vi "CENTRIOD DETECTION BEAMPOINTING.vi"(0 "Refnum in":T6=refnum, 4 "beam detection para":T4={"Filter"=1, "Filter Para"={"X Size"=5, "Y Size"=5, "% Tolerance"=1}, "detection method"=4, "smal para"=[{"Measurement Parameter"=35, "Range Lower Value"=0.0, "Range Upper Value"=500.0, "Range"=TRUE, "Measurement Type"=FALSE}], "Remove small Objects"=TRUE, "Restrict to round Objects"=TRUE} {"smal para"."Measurement Parameter" items=["Center of Mass X", "Center of Mass Y", "First Pixel X", "First Pixel Y", "Bounding Rect Left", "Bounding Rect Top", "Bounding Rect Right", "Bounding Rect Bottom", "Max Feret Diameter Start X", "Max Feret Diameter Start Y", "Max Feret Diameter End X", "Max Feret Diameter End Y", "Max Horiz. Segment Length Left", "Max Horiz. Segment Length Right", "Max Horiz. Segment Length Row", "-", "Bounding Rect Width", "Bounding Rect Height", "Bounding Rect Diagonal", "Perimeter", "Convex Hull Perimeter", "Holes' Perimeter", "Max Feret Diameter", "Equivalent Ellipse Major Axis", "Equivalent Ellipse Minor Axis", "Equivalent Ellipse Minor Axis (Feret)", "Equivalent Rect Long Side", "Equivalent Rect Short Side", "Equivalent Rect Diagonal", "Equivalent Rect Short Side (Feret)", "Average Horiz. Segment Length", "Average Vert. Segment Length", "Hydraulic Radius", "Waddel Disk Diameter", "-", "Area", "Holes' Area", "Particle & Holes' Area", "Convex Hull Area", "Image Area", "-", "Number of Holes", "Number of Horiz. Segments", "Number of Vert. Segments", "-", "Orientation", "Max Feret Diameter Orientation", "-", "% Area/Image Area", "% Area/(Particle & Holes' Area)", "Ratio of Equivalent Ellipse Axes", "Ratio of Equivalent Rect Sides", "-", "Elongation Factor", "Compactness Factor", "Heywood Circularity Factor", "Type Factor", "-", "Sum X", "Sum Y", "Sum XX", "Sum XY", "Sum YY", "Sum XXX", "Sum XXY", "Sum XYY", "Sum YYY", "-", "Moment of Inertia XX", "Moment of Inertia XY", "Moment of Inertia YY", "Moment of Inertia XXX", "Moment of Inertia XXY", "Moment of Inertia XYY", "Moment of Inertia YYY", "Norm. Moment of Inertia XX", "Norm. Moment of Inertia XY", "Norm. Moment of Inertia YY", "Norm. Moment of Inertia XXX", "Norm. Moment of Inertia XXY", "Norm. Moment of Inertia XYY", "Norm. Moment of Inertia YYY", "Hu Moment 1", "Hu Moment 2", "Hu Moment 3", "Hu Moment 4", "Hu Moment 5", "Hu Moment 6", "Hu Moment 7"]; "smal para"."Range Lower Value" format="%.2f"; "smal para"."Range Upper Value" format="%.2f"; "detection method" items=["clustering", "entropy", "metric", "moments", "inter-class variance"]; "Filter" items=["No Filter", "Median Filter", "Low Pass Filter"]}, 5 "error in (no error)":errorcluster) -> (8 "Bounding Rect":T7={"Left"=200.0, "Top"=222.0, "Right"=337.0, "Bottom"=354.0}, 11 "Particle Reports (Pixels)":T8(array[cluster])=[{"Area"=13217.0, "Number of Holes"=0.0, "Bounding Rect"={"Left"=200.0, "Top"=222.0, "Right"=337.0, "Bottom"=354.0}, "Center of Mass"={"X"=269.13989558901415, "Y"=287.03949459030036}, "Orientation"=28.32814462161336, "Dimensions"={"Width"=137.0, "Height"=132.0}}] {"Orientation" format="%.2f"; "Dimensions"."Height" format="%.2f"; "Dimensions"."Width" format="%.2f"; "Center of Mass"."Y" format="%.2f"; "Center of Mass"."X" format="%.2f"; "Bounding Rect"."Bottom" format="%.2f"; "Bounding Rect"."Right" format="%.2f"; "Bounding Rect"."Top" format="%.2f"; "Bounding Rect"."Left" format="%.2f"; "Number of Holes" format="%.2f"; "Area" format="%.2f"}, 13 "Area":dbl=13217.0, 14 "Refnum out":T6, 17 "Number of Particles":i32=1, 18 "Centriod":cluster{"X":dbl, "Y":dbl}={"X"=268.53924560546875, "Y"=286.7691955566406}, 19 "error out":errorcluster)   [LabVIEW 2013]
uses:
  <vilib>/vision/Image Controls.llb/IMAQ Image.ctl
  Ctrs/beam detection.ctl
  <vilib>/vision/Measure.llb/Edge Options.ctl
  <vilib>/vision/Measure.llb/Edge Polarity.ctl
  <vilib>/vision/NI_Vision_Development_Module.lvlib
panel:
  out "Circle Found":bool=TRUE
  in  "Options":T3={"Search  Direction"=1, "Edge Options"={"Edge Polarity"=2, "Kernel Size"=3, "Width"=3, "Minimum Edge Strength"=10.0, "Interpolation Type"=enum."Bilinear Fixed", "Data Processing Method"=enum."Average"}, "Show Search Area"=FALSE, "Show Search Lines"=FALSE, "Show Edges Found"=FALSE, "Show Result"=TRUE, "Search Area Color"=65280, "Search Lines Color"=255, "Edge Locations Color"=16776960, "Result Color"=3079978, "Overlay Group Name"=""} {"Search  Direction" items=["Outside to Inside", "Inside to Outside"]; "Edge Options"."Edge Polarity" items=["All Edges", "Rising Edges", "Falling Edges"]; "Edge Options"."Minimum Edge Strength" format="%.2f"; "Edge Options"."Width" step=2; "Edge Options"."Kernel Size" step=2}
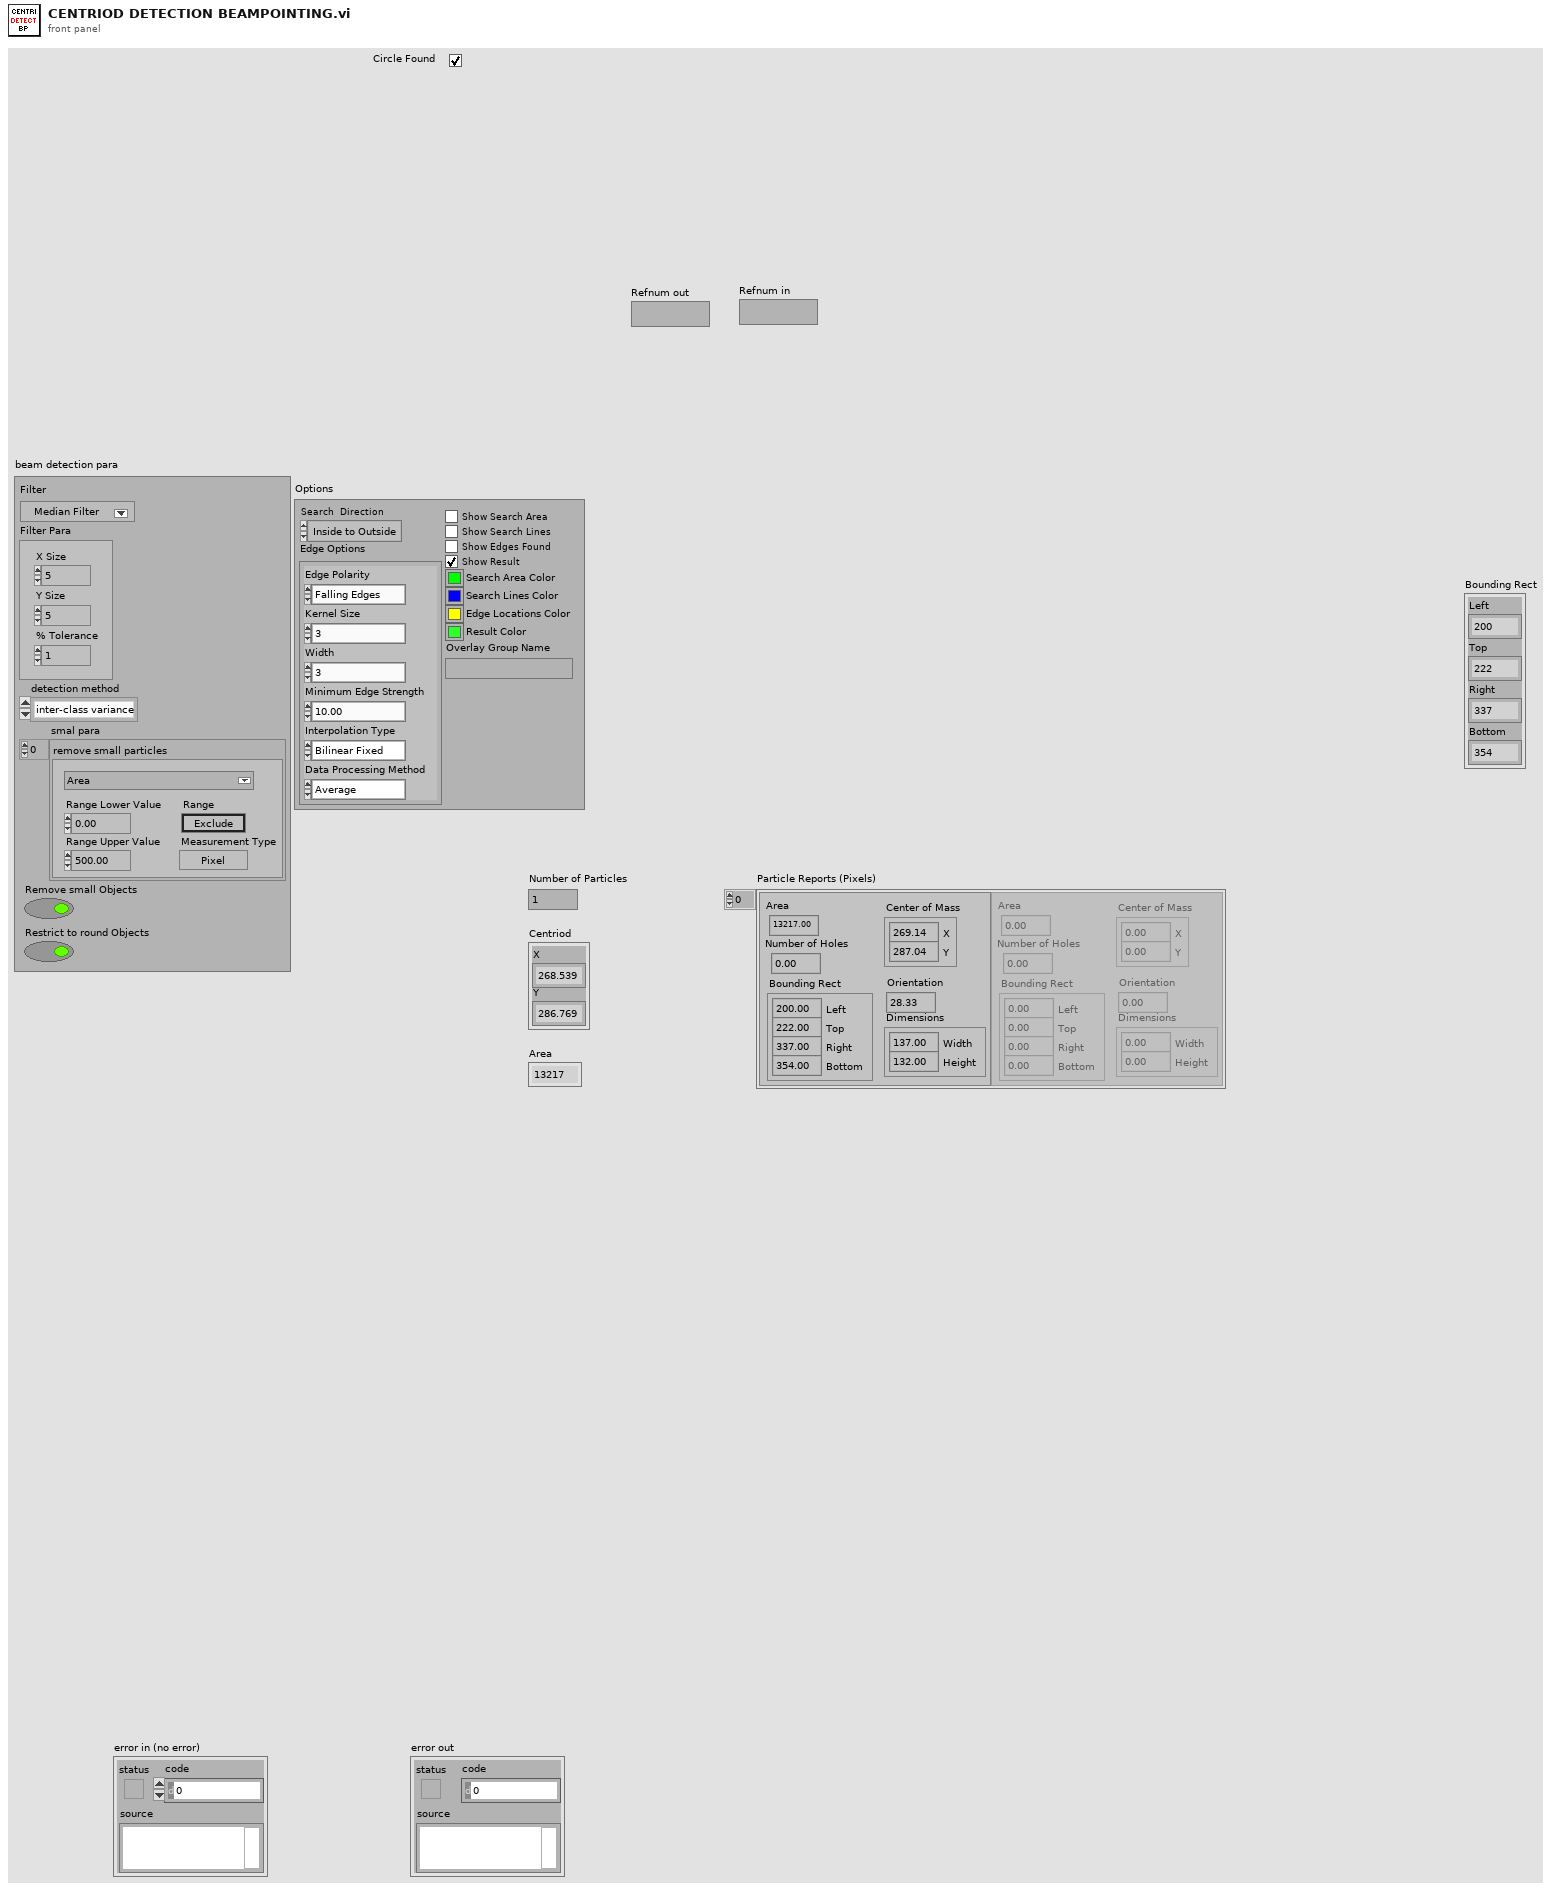
[diagram p1: front panel]
types:
  T1 = typedef "Edge Options.ctl" = cluster{"Edge Polarity":T2, "Kernel Size":u32, "Width":u32, "Minimum Edge Strength":sgl, "Interpolation Type":enum32{"Zero Order", "Bilinear", "Quadratic", "Cubic", "Bilinear Fixed"}, "Data Processing Method":enum32{"Average", "Median"}}
  T2 = typedef "Edge Polarity.ctl" = u32
  T3 = cluster{"Search  Direction":u32, "Edge Options":T1, "Show Search Area":bool, "Show Search Lines":bool, "Show Edges Found":bool, "Show Result":bool, "Search Area Color":u32, "Search Lines Color":u32, "Edge Locations Color":u32, "Result Color":u32, "Overlay Group Name":string}
  T4 = typedef "beam detection.ctl" = cluster{"Filter":u16, "Filter Para":cluster{"X Size":i32, "Y Size":i32, "% Tolerance":i32}, "detection method":i32, "smal para":cluster{"Measurement Parameter":T5, "Range Lower Value":dbl, "Range Upper Value":dbl, "Range":bool, "Measurement Type":bool}[], "Remove small Objects":bool, "Restrict to round Objects":bool}
  T5 = typedef "Particle Parameters" = i32
  T6 = typedef "IMAQ Image.ctl" = refnum<image>
  T7 = cluster{"Left":dbl, "Top":dbl, "Right":dbl, "Bottom":dbl}
  T8 = cluster{"Area":dbl, "Number of Holes":dbl, "Bounding Rect":cluster{"Left":dbl, "Top":dbl, "Right":dbl, "Bottom":dbl}, "Center of Mass":cluster{"X":dbl, "Y":dbl}, "Orientation":dbl, "Dimensions":cluster{"Width":dbl, "Height":dbl}}[]
  T9 = typedef "Image Type" = u32
  T10 = cluster{"X Size":i32, "Y Size":i32, "% Tolerance":i32}
  T11 = typedef "IMAQ Circle" = cluster{"Center X":i32, "Center Y":i32, "Inner Radius":i32, "Outer Radius":i32, "Start Angle":dbl, "End Angle":dbl}
  T12 = cluster{"Measurement Parameter":T5, "Range Lower Value":dbl, "Range Upper Value":dbl, "Range":bool, "Measurement Type":bool}[]
  T13 = cluster{"Area":dbl, "Number of Holes":dbl, "Bounding Rect":cluster{"Left":dbl, "Top":dbl, "Right":dbl, "Bottom":dbl}, "Center of Mass":cluster{"X":dbl, "Y":dbl}, "Orientation":dbl, "Dimensions":cluster{"Width":dbl, "Height":dbl}}
  T14 = typedef "ROI Descriptor" = cluster{"Global Rectangle":i32[], "Contours":cluster{"ID":enum32{"External", "Internal"}, "Type":u32, "Coordinates":i32[]}[]}
  T15 = cluster{"Center (Pixels)":cluster{"X":sgl, "Y":sgl}, "Radius (Pixels)":dbl, "Center (Real-World)":cluster{"X":sgl, "Y":sgl}, "Radius (Real-World)":dbl, "Roundness (Real-World)":dbl, "Average Strength":dbl, "Average SNR (dB)":dbl}
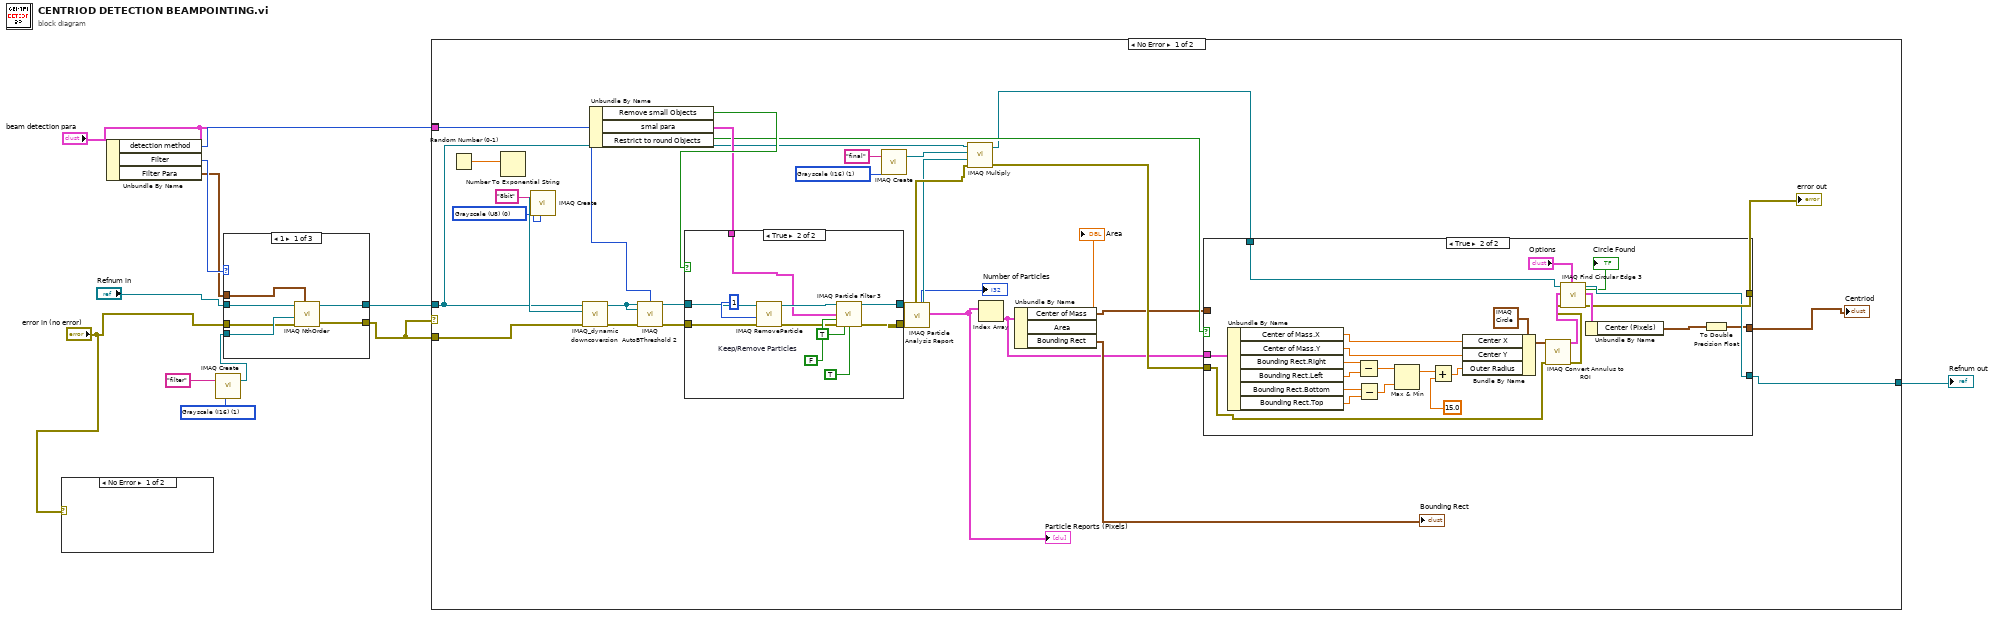
[diagram p0: block diagram]
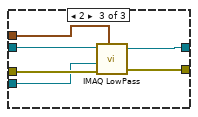
[diagram p7: hidden frame]
diagram:
  w12 = T9 1 items=["Grayscale (U8)", "Grayscale (I16)", "Grayscale (SGL)", "Complex (CSG)", "RGB (U32)", "HSL (U32)", "RGB (U64)", "Grayscale (U16)"] ("Image Type")
  n1 = case shown="No Error" "error in (no error)" {
    frame No Error {
    }
    frame Error {
    }
  }
  n2 = Unbundle By Name("beam detection para") -> ("detection method"=w9:i32, "Filter"=w10:u16, "Filter Para"=w8:T10)
  n3 = call "IMAQ Create"("Image Name"="filter", "Image Type"=w12) -> ("New Image"=w11:T6)  [unwired: 3 in, 1 out]
  n4 = case shown="1" w10 {
    tunnel: "error in (no error)" -> [w15 w19 w26]
    tunnel: "Refnum in" -> [w17 w20 w25]
    tunnel: w8 -> [w18 _ w24]
    tunnel: [w13 w20 w23] -> w5
    tunnel: w11 -> [w16 _ w22]
    tunnel: [w14 w19 w21] -> w2
    frame 1 {
      n5 = call "IMAQ NthOrder"("Image Src"=w17, "Size & Order #"=w18, "Image Dst"=w16, "error in (no error)"=w15) -> ("Image Dst Out"=w13:T6, "error out"=w14:errorcluster)  [unwired: 3 in]
    }
    frame 0, Default {
    }
    frame 2 {
      n6 = call "IMAQ LowPass"("Image Src"=w25, "Size & Tolerance"=w24, "Image Dst"=w22, "error in (no error)"=w26) -> ("Image Dst Out"=w23:T6, "error out"=w21:errorcluster)  [unwired: 3 in]
    }
  }
  n7 = case shown="No Error" w2 {
    tunnel: w2 -> [w57 _]
    tunnel: w9 -> [w44 _]
    tunnel: "beam detection para" -> [w43 _]
    tunnel: w5 -> [w33 w101]
    tunnel: [w27 w101] -> w4
    frame No Error {
      w53 = T9 0 items=["Grayscale (U8)", "Grayscale (I16)", "Grayscale (SGL)", "Complex (CSG)", "RGB (U32)", "HSL (U32)", "RGB (U64)", "Grayscale (U16)"] ("Image Type")
      w51 = T9 1 items=["Grayscale (U8)", "Grayscale (I16)", "Grayscale (SGL)", "Complex (CSG)", "RGB (U32)", "HSL (U32)", "RGB (U64)", "Grayscale (U16)"] ("Image Type")
      n8 = Random Number (0-1)() -> (number: 0 to 1=w40:dbl)
      n9 = Number To Exponential String(number=w40) -> ()  [unwired: 3 in, 1 out]
      n10 = call "IMAQ Create"("Image Name"="8bit", "Image Type"=w53) -> ("New Image"=w54:T6)  [unwired: 3 in, 1 out]
      n11 = call "IMAQ_dynamic downcoversion.vi"("error in (no error)"=w57, "Image Dst"=w54, "Image Src"=w33) -> ("error out"=w56:errorcluster, "Image Out"=w55:T6)  [unwired: 7 in]
      n12 = Unbundle By Name(w43) -> ("Remove small Objects"=w42:bool, "smal para"=w41:T12, "Restrict to round Objects"=w38:bool)
      n13 = call "IMAQ AutoBThreshold 2"("Image Src"=w55, "Method (clustering)"=w44, "Image Dst"=w55, "error in (no error)"=w56) -> ("Image Dst Out"=w46:T6, "error out"=w47:errorcluster)  [unwired: 9 in, 1 out]
      n14 = case shown="True" w42 {
        tunnel: [w89 w96] -> w48
        tunnel: [w88 w95] -> w49
        tunnel: w46 -> [w89 w94]
        tunnel: w47 -> [w88 w93]
        tunnel: w41 -> [_ w91]
        frame False {
        }
        frame True {
          w100 = FALSE  # Keep/Remove Particles
          n15 = call "IMAQ RemoveParticle"("error in (no error)"=w93, "Number of Erosion"=1 ("Numeric"), "Image Src"=w94) -> ("error out"=w97:errorcluster, "Image Dst Out"=w98:T6)  [unwired: 4 in, 3 out]
          n16 = call "IMAQ Particle Filter 3"("Image Src"=w98, "Selection Values"=w91, "Keep/Remove Particles (F)"=w100, "error in (no error)"=w97, "Reject Border? (F)"=TRUE, "Fill Holes? (F)"=TRUE) -> ("Image Dst Out"=w96:T6, "error out"=w95:errorcluster)  [unwired: 3 in, 5 out]
        }
      }
      n17 = call "IMAQ Create"("Image Name"="final", "Image Type"=w51) -> ("New Image"=w52:T6)  [unwired: 3 in, 1 out]
      n18 = call "IMAQ Particle Analysis Report"("error in (no error)"=w49, "Image"=w48) -> ("error out"=w58:errorcluster, "Particle Reports (Pixels)"=w32:T8, "Image Out (duplicate)"=w50:T6, "Number of Particles"=→"Number of Particles":i32)  [unwired: 4 in, 2 out]
      "Particle Reports (Pixels)" <- w32
      n19 = call "IMAQ Multiply"("Image Src A"=w33, "Image Dst"=w52, "Image Src B"=w50, "error in (no error)"=w58) -> ("Image Dst Out"=w30:T6, "error out"=w37:errorcluster)  [unwired: 3 in]
      n20 = Index Array(array=w32) -> (element=w31:T13)  [unwired: 1 in]
      n21 = Unbundle By Name(w31) -> ("Center of Mass"=w29:cluster{"X":dbl, "Y":dbl}, "Area"=→"Area":dbl, "Bounding Rect"=→"Bounding Rect":T7)
      n22 = case shown="True" w38 {
        tunnel: w30 -> [w60 w87]
        tunnel: [w62 w80] -> w28
        tunnel: w29 -> [w62 _]
        tunnel: w37 -> [w61 w74]
        tunnel: [w61 w84] -> w36
        tunnel: [w60 w83] -> w27
        tunnel: w31 -> [_ w77]
        frame False {
        }
        frame True {
          n23 = Unbundle By Name(w77) -> ("Center of Mass.X"=w64:dbl, "Center of Mass.Y"=w63:dbl, "Bounding Rect.Right"=w69:dbl, "Bounding Rect.Left"=w68:dbl, "Bounding Rect.Bottom"=w67:dbl, "Bounding Rect.Top"=w66:dbl)
          n24 = Subtract(x=w69, y=w68) -> (x-y=w70:dbl)
          n25 = Subtract(x=w67, y=w66) -> (x-y=w71:dbl)
          n26 = Max & Min(x=w70, y=w71) -> (max(x,y)=w72:dbl)  [unwired: 1 out]
          n27 = Add(x=w72, y=15.0) -> (x+y=w65:dbl)
          n28 = Bundle By Name(cluster=T11 {"Center X"=0, "Center Y"=0, "Inner Radius"=0, "Outer Radius"=0, "Start Angle"=0.0, "End Angle"=360.0} ("Annulus"), "Center X"=w64, "Center Y"=w63, "Outer Radius"=w65) -> (w78:T11)
          n29 = call "IMAQ Convert Annulus to ROI"("error in (no error)"=w74, "Annulus"=w78) -> ("error out"=w75:errorcluster, "ROI Descriptor"=w76:T14)  [unwired: 7 in]
          n30 = call "IMAQ Find Circular Edge 3"("Options"="Options", "error in (no error)"=w75, "ROI Descriptor"=w76, "Image"=w87) -> ("error out"=w84:errorcluster, "Fitted Circle"=w85:T15, "Image Out"=w83:T6, "Circle Found"=→"Circle Found":bool)  [unwired: 3 in, 1 out]
          n31 = Unbundle By Name(w85) -> ("Center (Pixels)"=w81:cluster{"X":sgl, "Y":sgl})
          n32 = To Double Precision Float(number=w81) -> (double precision float=w80:cluster{"X":dbl, "Y":dbl})
        }
      }
      "error out" <- w36
      "Centriod" <- w28
    }
    frame Error {
    }
  }
  "Refnum out" <- w4
